vi "TEST-Get DataType Description String.vi"() -> ()   [LabVIEW 2017]
uses:
  test.lvclass
panel:
  out "Type 16":string
  out "Type 15":string
  out "Type 14":string
  out "Type 12":string
  out "Variant":variant
  out "Type 11":string
  out "Type 10":string
  out "Type 9":string
  out "Type 8":string
  out "Type 7":string
  out "Type 6":string
  out "Type 5":string
  out "Type 4":string
  out "Type 3":string
  out "Type 2":string
  out "Type":string
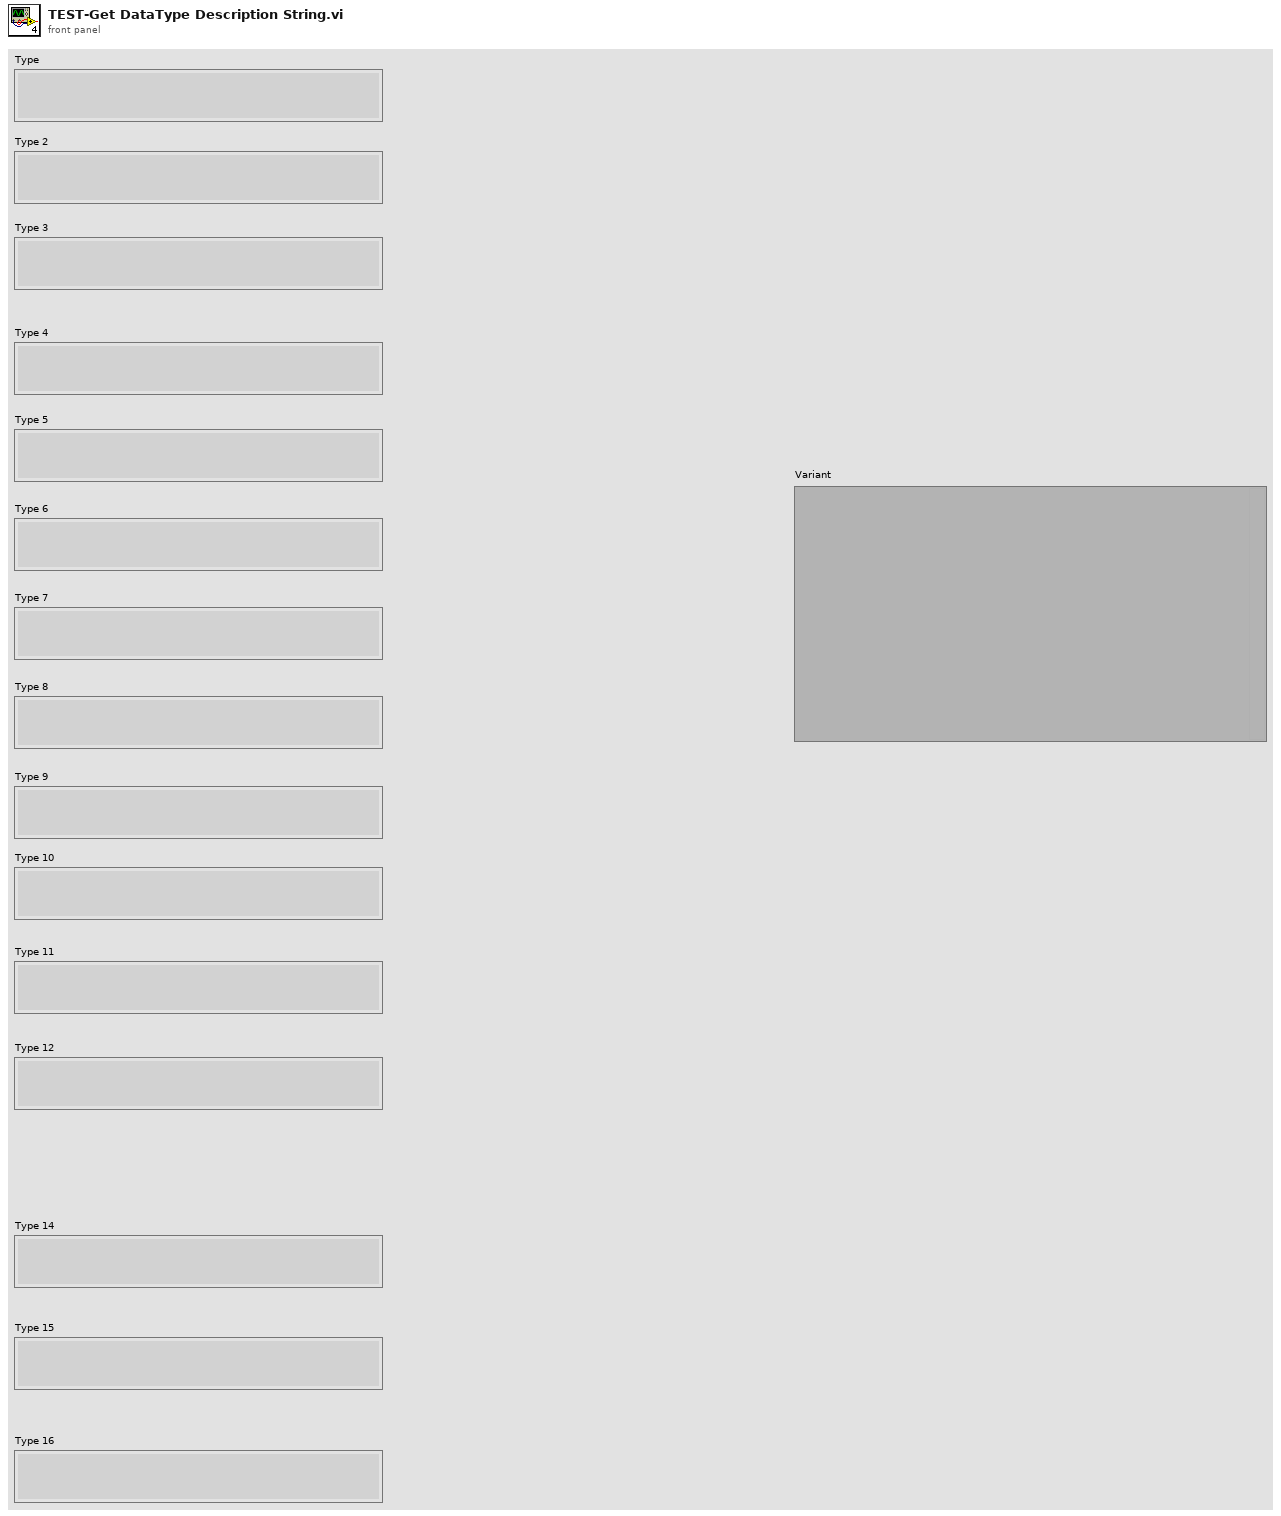
[diagram p1: front panel]
types:
  T1 = cluster{"status":bool, "code":i32, "source":string, "error in (no error)":errorcluster, "test.lvclass":refnum<class "test.lvclass">}[]
  T2 = cluster{"status":bool, "code":i32, "source":string, "error in (no error)":errorcluster, "test.lvclass":refnum<class "test.lvclass">, "aa":refnum<k1>}
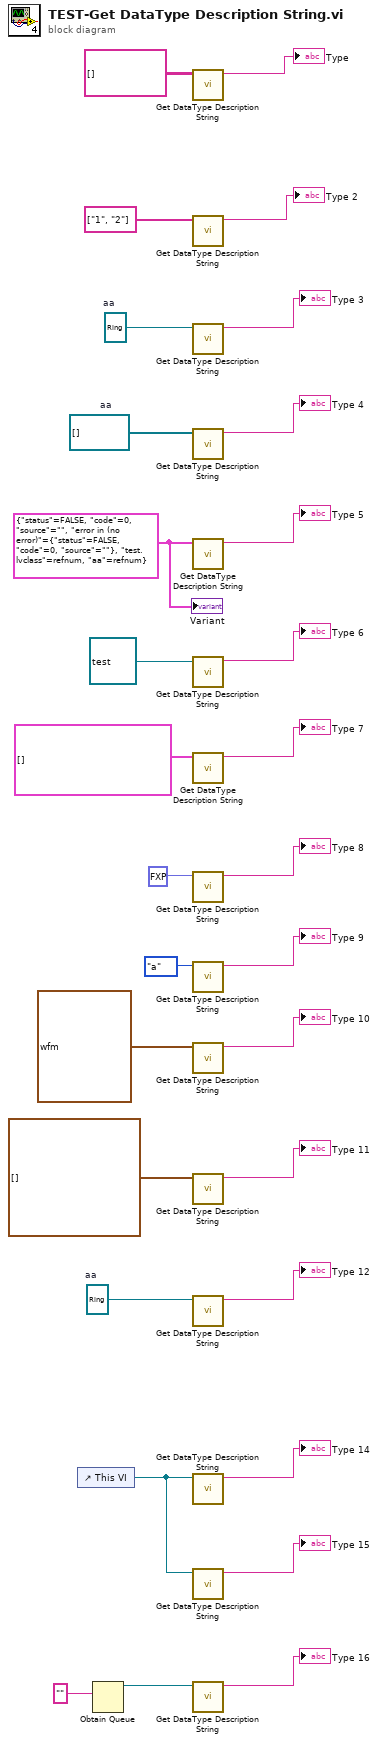
[diagram p0: block diagram]
diagram:
  w7 = refnum<k1> refnum  # aa
  w9 = T2 {"status"=FALSE, "code"=0, "source"="", "error in (no error)"={"status"=FALSE, "code"=0, "source"=""}, "test.lvclass"=refnum, "aa"=refnum} ("error in (no error)")
  w23 = refnum<k1>[] []  # aa
  w28 = refnum<k1> refnum  # aa
  n1 = control-ref of="This VI"() -> (w1:refnum<vi>)
  n2 = Obtain Queue(element data type="") -> (queue out=w2:refnum<queue>)  [unwired: 4 in, 2 out]
  n3 = call "Get DataType Description String.vi"("Variant"=string[][] []) -> ("String"=→"Type":string)  [unwired: 9 in, 1 out]
  n4 = call "Get DataType Description String.vi"("Variant"=string[] ["1", "2"]) -> ("String"=→"Type 2":string)  [unwired: 9 in, 1 out]
  n5 = call "Get DataType Description String.vi"("Variant"=w28) -> ("String"=→"Type 3":string)  [unwired: 9 in, 1 out]
  n6 = call "Get DataType Description String.vi"("Variant"=w23) -> ("String"=→"Type 4":string)  [unwired: 9 in, 1 out]
  n7 = call "Get DataType Description String.vi"("Variant"=w9) -> ("String"=→"Type 5":string)  [unwired: 9 in, 1 out]
  n8 = call "Get DataType Description String.vi"("Variant"=refnum<class "test.lvclass"> refnum ("test.lvclass")) -> ("String"=→"Type 6":string)  [unwired: 9 in, 1 out]
  n9 = call "Get DataType Description String.vi"("Variant"=T1 [] ("error in (no error)")) -> ("String"=→"Type 7":string)  [unwired: 9 in, 1 out]
  n10 = call "Get DataType Description String.vi"("Variant"=fxp<+/-,4,8> 0.0) -> ("String"=→"Type 8":string)  [unwired: 9 in, 1 out]
  n11 = call "Get DataType Description String.vi"("Variant"=enum32{"a", "b", "c", "d"}."a") -> ("String"=→"Type 9":string)  [unwired: 9 in, 1 out]
  n12 = call "Get DataType Description String.vi"("Variant"=waveform(dbl) {"t0"=timestamp(0 s since 1904-01-01), "dt"=1.0, "Y"=[]} ("Waveform")) -> ("String"=→"Type 10":string)  [unwired: 9 in, 1 out]
  n13 = call "Get DataType Description String.vi"("Variant"=waveform(u16)[] []) -> ("String"=→"Type 11":string)  [unwired: 9 in, 1 out]
  n14 = call "Get DataType Description String.vi"("Variant"=w7) -> ("String"=→"Type 12":string)  [unwired: 9 in, 1 out]
  n15 = call "Get DataType Description String.vi"("Variant"=w1) -> ("String"=→"Type 14":string)  [unwired: 9 in, 1 out]
  n16 = call "Get DataType Description String.vi"("Variant"=w1) -> ("String"=→"Type 15":string)  [unwired: 9 in, 1 out]
  n17 = call "Get DataType Description String.vi"("Variant"=w2) -> ("String"=→"Type 16":string)  [unwired: 9 in, 1 out]
  "Variant" <- w9
